vi "ERIO RT Distribute Alarms-Notifications.vi"(6 "Supervisory Variables In":T5={"Alarm Threshold"=0.0, "Shutdown"=FALSE, "Enable SNS Alarm"=FALSE, "Enable SNS Stage Notification"=FALSE, "Enable SQS Notification"=FALSE, "Enable S3 TDMS Signal Capture"=FALSE, "Enable SystemLink Signal Capture"=FALSE, "Capture Signal"=FALSE, "Server Update"=FALSE, "AWS Access Key"="AKIAINLDO2Y2PDFEWDOQ", "AWS Secret Key"="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", "Phone Number"="+15037066913", "Region"=enum."us-west-2", "AWS SQS Queue"="mynicloud-demotest2", "AWS S3 Bucket"="mynicloud-demotest2"}, 7 "RT State In":T2, 8 "error in (no error)":errorcluster, 9 "AWS Variables In":T7, 10 "Alarm-Notifier":T1=enum."Into Shutdown", 11 "EEISysLink.lvclass In":refnum<class "EEISysLink.lvclass">) -> (0 "error out":errorcluster, 1 "AWS Variables Out":T7, 3 "EEISysLink.lvclass Out":refnum<class "EEISysLink.lvclass">, 4 "Supervisory Variables Out":T5={"Alarm Threshold"=0.0, "Shutdown"=FALSE, "Enable SNS Alarm"=FALSE, "Enable SNS Stage Notification"=FALSE, "Enable SQS Notification"=FALSE, "Enable S3 TDMS Signal Capture"=FALSE, "Enable SystemLink Signal Capture"=FALSE, "Capture Signal"=FALSE, "Server Update"=FALSE, "AWS Access Key"="AKIAINLDO2Y2PDFEWDOQ", "AWS Secret Key"="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", "Phone Number"="+15037066913", "Region"=enum."us-west-2", "AWS SQS Queue"="mynicloud-demotest2", "AWS S3 Bucket"="mynicloud-demotest2"}, 5 "RT State Out":T2)   [LabVIEW 2017]
doc: "An alarm or notification event occurred. Distribute to enabled destinations.\n\nJames Tillett P.E.\nEndeavor Engineering Inc.\nwww.endeavoreng.com"
uses:
  Class EEISysLink/EEISysLink.lvclass
  Controls/ERIO AWS Toolkit Variables.ctl
  <vilib>/AWS Toolkit/SQS/Queue/Queue.lvclass
  <vilib>/AWS Toolkit/SNS/Phone Number/Phone Number.lvclass
  <vilib>/AWS Toolkit/S3/Bucket/Bucket.lvclass
  Controls/ERIO Supervisory Variables.ctl
  <vilib>/AWS Toolkit/Core/HTTP Request/Region.ctl
  Controls/ERIO RT State Variables.ctl
  Controls/ERIO SystemStates.ctl
  Controls/ERIO Queue Data.ctl
  Controls/ERIO Worker Variables.ctl
  Controls/ERIO Alarm-Notifier Action.ctl
  <vilib>/Utility/error.llb/Error Cluster From Error Code.vi
  <vilib>/rvi/errors/niLvFpgaAdjustHostInterfaceError.vi
  <vilib>/rvi/interface/nirviReadWriteControl/nirviReadWriteControl.xnode
  NiFpgaLv.dll
  <vilib>/rvi/interface/Simulation/niFpgaSimulationCallBeginRW.vi
  <vilib>/AWS Toolkit/Core/HTTP Request/HTTP Request.lvclass
panel:
  out "Last Notification":string
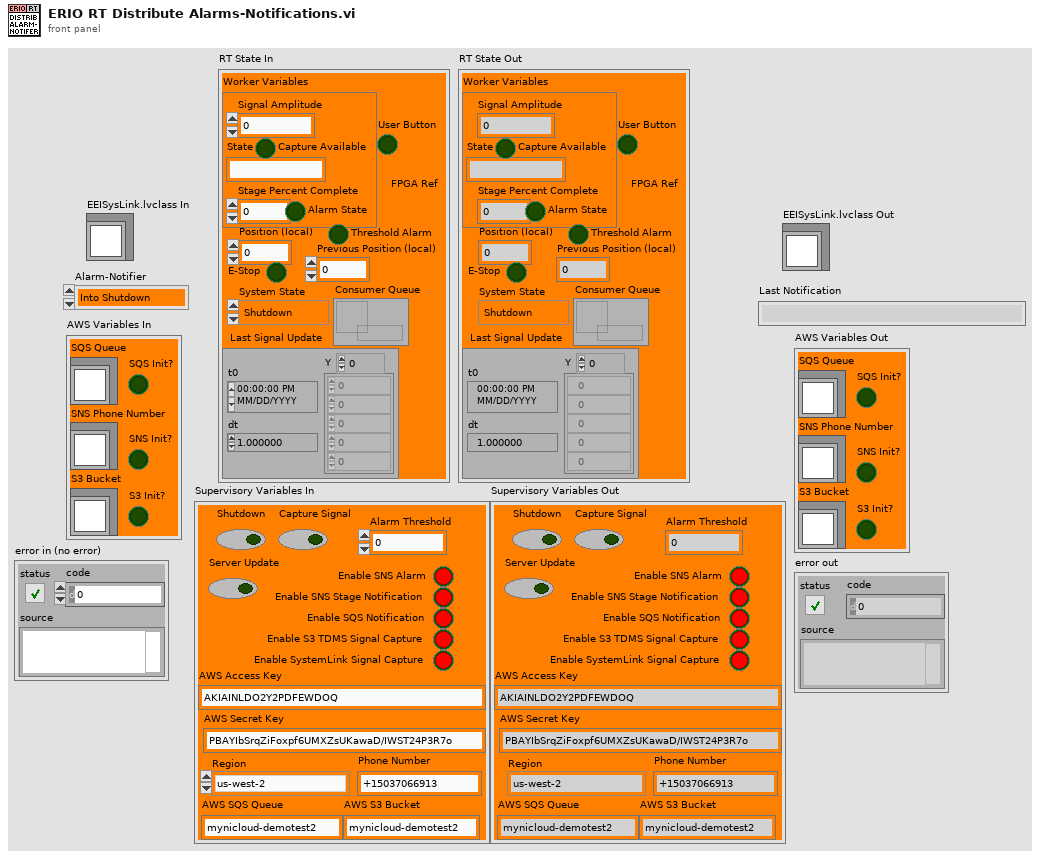
[diagram p1: front panel]
types:
  T1 = typedef "ERIO Alarm-Notifier Action.ctl" = enum16{"No Action", "Threshold Alarm", "Into Stage 1", "Into Stage 2", "Into Stage 3", "Into Shutdown", "Into Process Reset", "Into E-STOP", "User Button"}
  T2 = typedef "ERIO RT State Variables.ctl" = cluster{"Position (local)":i16, "E-Stop":bool, "System State":T3, "FPGA Ref":refnum<k20>, "Previous Position (local)":i16, "Consumer Queue":refnum<queue>, "Worker Variables":T4, "Threshold Alarm":bool, "User Button":bool, "Last Signal Update":waveform(dbl)}
  T3 = typedef "ERIO SystemStates.ctl" = enum16{"Shutdown", "E-STOP", "Reset Process", "Stage 1", "Stage 2", "Stage 3", "Alarm State"}
  T4 = typedef "ERIO Worker Variables.ctl" = cluster{"Signal Amplitude":dbl, "State":string, "Stage Percent Complete":dbl, "Alarm State":bool, "Capture Available":bool}
  T5 = typedef "ERIO Supervisory Variables.ctl" = cluster{"Alarm Threshold":dbl, "Shutdown":bool, "Enable SNS Alarm":bool, "Enable SNS Stage Notification":bool, "Enable SQS Notification":bool, "Enable S3 TDMS Signal Capture":bool, "Enable SystemLink Signal Capture":bool, "Capture Signal":bool, "Server Update":bool, "AWS Access Key":string, "AWS Secret Key":string, "Phone Number":string, "Region":T6, "AWS SQS Queue":string, "AWS S3 Bucket":string}
  T6 = typedef "NI_AWS_Core.lvlib/HTTP Request.lvclass/Region.ctl" = enum16{"us-east-1", "us-east-2", "us-west-1", "us-west-2", "ap-northeast-1", "ap-northeast-2", "ap-southeast-1", "ap-southeast-2", "ca-central-1", "eu-central-1", "eu-west-1", "eu-west-2", "sa-east-1"}
  T7 = typedef "ERIO AWS Toolkit Variables.ctl" = cluster{"SQS Queue":refnum<class "Queue.lvclass">, "SNS Phone Number":refnum<class "Phone Number.lvclass">, "S3 Bucket":refnum<class "Bucket.lvclass">, "SQS Init?":bool, "S3 Init?":bool, "SNS Init?":bool}
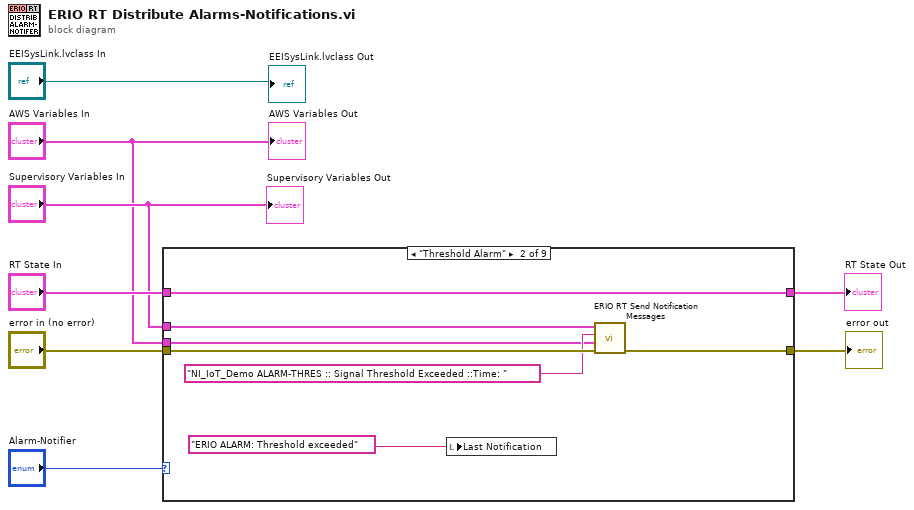
[diagram p0: block diagram]
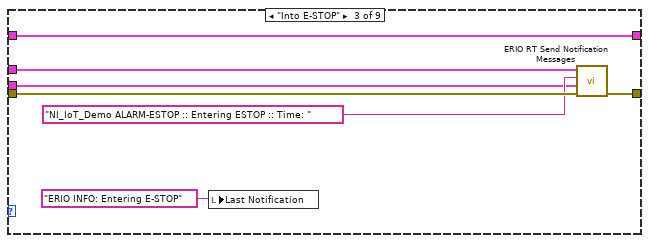
[diagram p3: hidden frame]
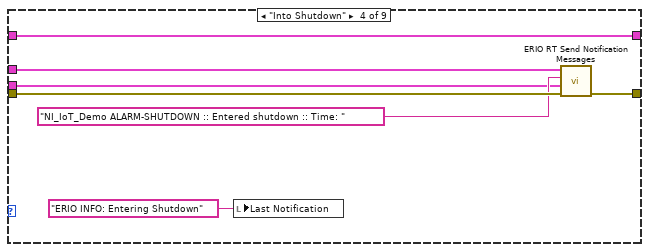
[diagram p4: hidden frame]
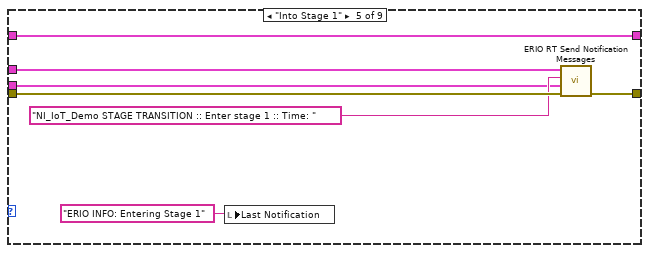
[diagram p5: hidden frame]
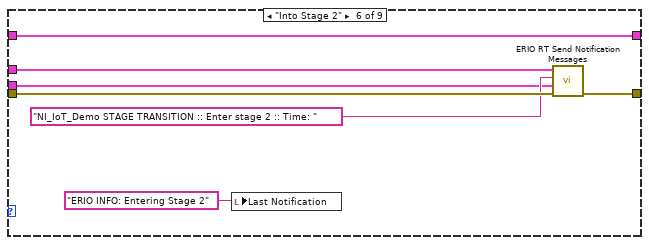
[diagram p6: hidden frame]
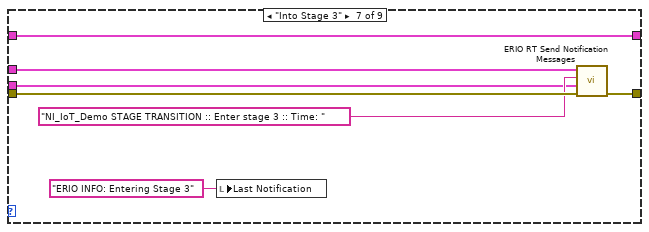
[diagram p7: hidden frame]
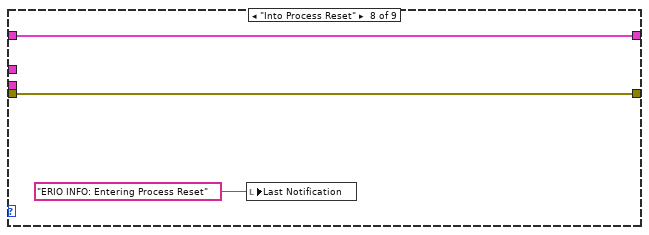
[diagram p8: hidden frame]
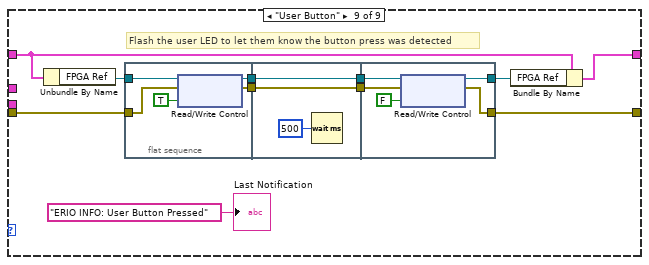
[diagram p9: hidden frame]
diagram:
  n1 = case shown="\"Threshold Alarm\"" "Alarm-Notifier" {
    tunnel: "RT State In" -> [w9 w16 w24 w31 w38 w45 w52 w54 w59]
    tunnel: "error in (no error)" -> [w10 w15 w23 w30 w37 w44 w51 w53 w64]
    tunnel: [w10 w14 w22 w29 w36 w43 w50 w53 w56] -> w4
    tunnel: [w9 w16 w24 w31 w38 w45 w52 w54 w57] -> w3
    tunnel: "Supervisory Variables In" -> [_ w12 w20 w27 w34 w41 w48 _ _]
    tunnel: "AWS Variables In" -> [_ w11 w18 w25 w32 w39 w46 _ _]
    frame "No Action", Default {
    }
    frame "Threshold Alarm" {
      n2 = local write "Last Notification"("ERIO ALARM: Threshold exceeded") -> ()
      n3 = call "ERIO RT Send Notification Messages.vi"("error in (no error)"=w15, "AWS Variables In"=w11, "Message Body"="NI_IoT_Demo ALARM-THRES :: Signal Threshold Exceeded ::Time: ", "Supervisory Variables In"=w12) -> ("error out"=w14:errorcluster)  [unwired: 6 in, 1 out]
    }
    frame "Into E-STOP" {
      n4 = local write "Last Notification"("ERIO INFO: Entering E-STOP") -> ()
      n5 = call "ERIO RT Send Notification Messages.vi"("error in (no error)"=w23, "AWS Variables In"=w18, "Message Body"="NI_IoT_Demo ALARM-ESTOP :: Entering ESTOP :: Time: ", "Supervisory Variables In"=w20) -> ("error out"=w22:errorcluster)  [unwired: 6 in, 1 out]
    }
    frame "Into Shutdown" {
      n6 = local write "Last Notification"("ERIO INFO: Entering Shutdown") -> ()
      n7 = call "ERIO RT Send Notification Messages.vi"("error in (no error)"=w30, "AWS Variables In"=w25, "Message Body"="NI_IoT_Demo ALARM-SHUTDOWN :: Entered shutdown :: Time: ", "Supervisory Variables In"=w27) -> ("error out"=w29:errorcluster)  [unwired: 6 in, 1 out]
    }
    frame "Into Stage 1" {
      n8 = local write "Last Notification"("ERIO INFO: Entering Stage 1") -> ()
      n9 = call "ERIO RT Send Notification Messages.vi"("error in (no error)"=w37, "AWS Variables In"=w32, "Message Body"="NI_IoT_Demo STAGE TRANSITION :: Enter stage 1 :: Time: ", "Supervisory Variables In"=w34) -> ("error out"=w36:errorcluster)  [unwired: 6 in, 1 out]
    }
    frame "Into Stage 2" {
      n10 = local write "Last Notification"("ERIO INFO: Entering Stage 2") -> ()
      n11 = call "ERIO RT Send Notification Messages.vi"("error in (no error)"=w44, "AWS Variables In"=w39, "Message Body"="NI_IoT_Demo STAGE TRANSITION :: Enter stage 2 :: Time: ", "Supervisory Variables In"=w41) -> ("error out"=w43:errorcluster)  [unwired: 6 in, 1 out]
    }
    frame "Into Stage 3" {
      n12 = local write "Last Notification"("ERIO INFO: Entering Stage 3") -> ()
      n13 = call "ERIO RT Send Notification Messages.vi"("error in (no error)"=w51, "AWS Variables In"=w46, "Message Body"="NI_IoT_Demo STAGE TRANSITION :: Enter stage 3 :: Time: ", "Supervisory Variables In"=w48) -> ("error out"=w50:errorcluster)  [unwired: 6 in, 1 out]
    }
    frame "Into Process Reset" {
      n14 = local write "Last Notification"("ERIO INFO: Entering Process Reset") -> ()
    }
    frame "User Button" {
      # "Flash the user LED to let them know the button press was detected"
      n15 = Unbundle By Name(w59) -> ("FPGA Ref"=w65:refnum<k20>)
      n16 = flat-sequence {
        tunnel: w65 -> [w71]
        tunnel: w64 -> [w69]
        tunnel: [w68] -> w62
        tunnel: [w67] -> w61
        tunnel: [w73] -> w63
        tunnel: w62 -> [w73]
        tunnel: w61 -> [w72]
        tunnel: [w72] -> w60
        tunnel: w63 -> [w78]
        tunnel: w60 -> [w77]
        tunnel: [w76] -> w58
        tunnel: [w75] -> w56
        frame #0 {
          n17 = xnode "Read/Write Control"("FPGA VI Reference In"=w71, "error in"=w69, "User LED"=TRUE) -> ("FPGA VI Reference Out"=w68:refnum<k20>, "error out"=w67:errorcluster)
        }
        frame #1 {
          n18 = Wait (ms)(milliseconds to wait=u32 500) -> ()  [unwired: 1 out]
        }
        frame #2 {
          n19 = xnode "Read/Write Control"("FPGA VI Reference In"=w78, "error in"=w77, "User LED"=FALSE) -> ("FPGA VI Reference Out"=w76:refnum<k20>, "error out"=w75:errorcluster)
        }
      }
      n20 = Bundle By Name(cluster=w59, "FPGA Ref"=w58) -> (w57:T2)
      "Last Notification" <- "ERIO INFO: User Button Pressed"
    }
  }
  "error out" <- w4
  "RT State Out" <- w3
  "EEISysLink.lvclass Out" <- "EEISysLink.lvclass In"
  "AWS Variables Out" <- "AWS Variables In"
  "Supervisory Variables Out" <- "Supervisory Variables In"
